vi "FACTORIAL OF A GIVE NUMBER USING WHILE.vi"() -> ()   [LabVIEW 2024]
panel:
  out "Output":dbl
  in  "Input":dbl
  in  "Constant":dbl
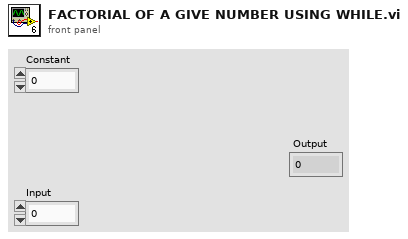
[diagram p1: front panel]
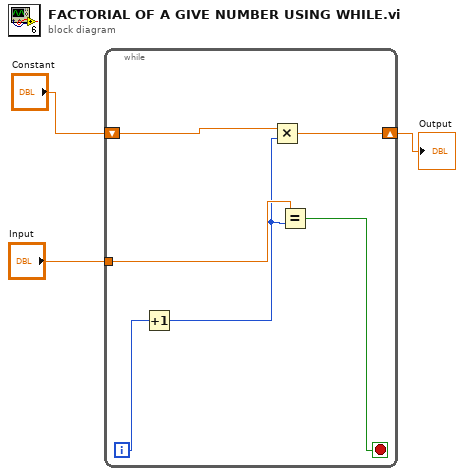
[diagram p0: block diagram]
diagram:
  n1 = while {
    tunnel: "Input" -> [w7]
    shift-right: [w9] -> w3
    shift-left: "Constant" -> [w8]
    i -> [w5]
    stop <- w4 stop-if-true
    n2 = Increment(x=w5) -> (x+1=w6:i32)
    n3 = Multiply(x=w8, y=w6) -> (x*y=w9:dbl)
    n4 = Equal?(x=w7, y=w6) -> (x = y?=w4:bool)
  }
  "Output" <- w3
